vi "DB Create Tables.vi"(8 "error in (no error)":errorcluster, 9 "Create Table":T3={"table"="", "column information"=[], "primary key (-1)"=-1, "use file? (F)"=FALSE}, 11 "SQLite Database in":refnum<class "SQLite Database.lvclass">) -> (0 "error out":errorcluster, 3 "SQLite Database out":refnum<class "SQLite Database.lvclass">)   [LabVIEW 2023, in "HardwareAbstractionLayer_LVOOP.lvlib" / "SQLite Database.lvclass"]
uses:
  SQLite Database.lvclass
  <vilib>/addons/database/Auxilliary.llb/DB Tools Column Info.ctl
  <vilib>/addons/database/Auxilliary.llb/DB Tools DataTypes.ctl
  <vilib>/addons/database/NI_Database_API.lvlib
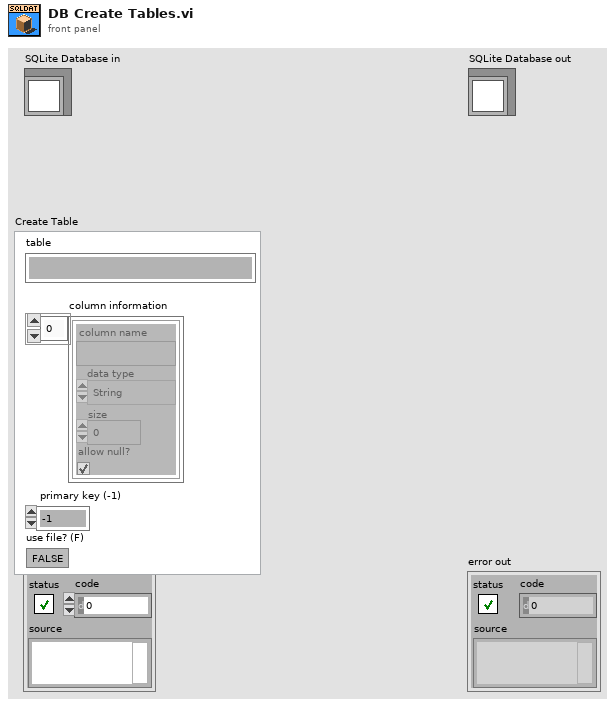
[diagram p1: front panel]
types:
  T1 = typedef "NI_Database_API.lvlib/DB Tools Column Info.ctl" = cluster{"column name":string, "data type":T2, "size":i32, "allow null?":bool}
  T2 = typedef "NI_Database_API.lvlib/DB Tools DataTypes.ctl" = enum16{"String", "Long (I32)", "Single (SGL)", "Double (DBL)", "Date/Time", "Binary"}
  T3 = cluster{"table":string, "column information":T1[], "primary key (-1)":i32, "use file? (F)":bool}
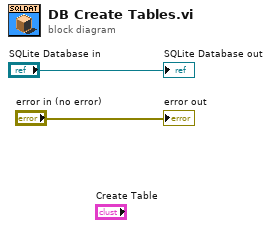
[diagram p0: block diagram]
diagram:
  "error out" <- "error in (no error)"
  "SQLite Database out" <- "SQLite Database in"
